vi "Magnet Gap Tester (RT).vi"() -> ()   [LabVIEW 2013]
uses:
  Controls/i2c_state.ctl
  Controls/Host_I2CBus_Options.ctl
  Controls/i2c_Protocol_Timing.ctl
  <vilib>/Analysis/polynomials.llb/Scalar Polynomial Evaluation (DBL).vi
  <vilib>/Utility/error.llb/Error Cluster From Error Code.vi
  <vilib>/rvi/errors/niLvFpgaAdjustHostInterfaceError.vi
  <vilib>/Analysis/polynomials.llb/1D Polynomial Evaluation (DBL).vi
  <vilib>/rvi/interface/common/niFpgaWaitOnOcc.vi
  <userlib>/_MGI/1D Array/MGI Average/MGI Average (DBL[]).vi
  <vilib>/rvi/interface/nirviReadWriteControl/nirviReadWriteControl.xnode
  Controls/FPGA_Reference.ctl
  FPGA Bitfiles/TIsbRIO_FPGATarget_TISensoredBLDC(F_DyXSZt47tvg.lvbitx
  FPGA/TI Sensored BLDC (FPGA).vi
  <vilib>/rvi/interface/nirviMethod/nirviMethod.xnode
  <vilib>/rvi/errors/niLvFpgaMergeErrorWithErrorCode.vi
  <vilib>/Analysis/NI_AALPro.lvlib
  <vilib>/FPGAPlugInAG/sbRIO-9626/niLvFpga_ReadFifo_sbRIO-9626.vi
  NiFpgaLv.dll
panel:
  out "Re-Cal (Hall)":dbl[](array[numeric])
  out "Re-Cal (Encoder)":dbl[](array[numeric])
  out "FWD Accuracy (%)":dbl
  out "REV Accuracy (%)":dbl
  out "REV Non-Linearity (%)":dbl=0.15612299232428833
  out "FWD Non-Linearity (%)":dbl=0.23166191431116404
  out "Max Hysteresis (%)":dbl=1.342957067692166
  out "Average Hysteresis (%)":dbl=0.6751303305956703
  out "Magnetic Field":u16=445
  out "Hall Pos (deg)":dbl=250.14822489420567
  out "ENC Pos (deg)":dbl=251.61773088654434
  in  "Motor Stop Offset":i32
  in  "REV Limit":dbl=90.0
  in  "FWD Limit":dbl=270.0
  out "XY Graph":cluster{dbl[], dbl[]}[](graph)=[{array[264 elements], array[264 elements]}, {array[264 elements], array[264 elements]}, {array[3405 elements], array[3405 elements]}, {array[3405 elements], array[3405 elements]}, {array[3405 elements], array[3405 elements]}, {[15041.030640668523, 5013.676880222842], [15041.030640668523, 5013.676880222842]}]
  out "Hall Elements":u32=3405
  out "Encoder Elements":u32=3405
  out "REV OUT":bool
  out "FWD OUT":bool
  in  "Reverse":bool
  in  "Forward":bool
  out "AI0":fxp<+/-,24,5>=2.0473861694335938
  out "ENC Pos (Counts)":i32=14017
  out "AI Loop Actual":u32=17
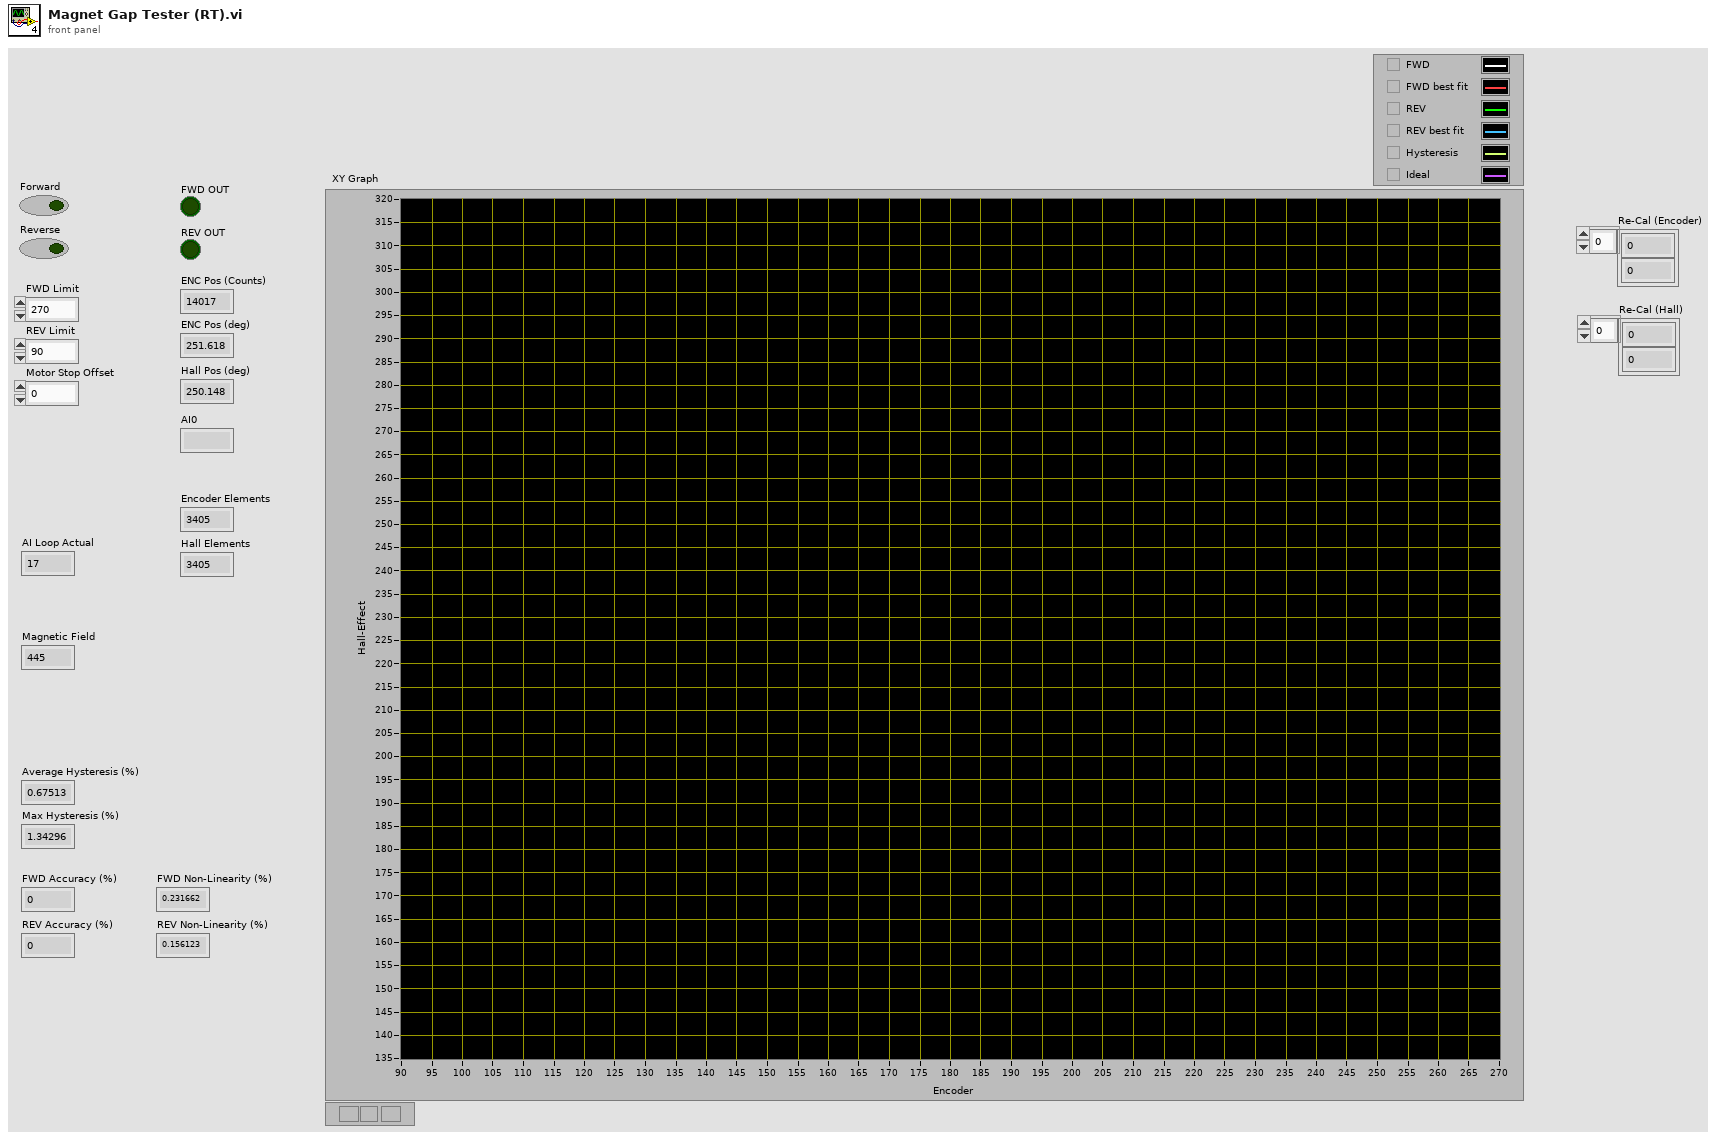
[diagram p1: front panel]
types:
  T1 = typedef "i2c_Protocol_Timing.ctl" = cluster{"SCL Period (Ticks)":u32, "TransmitDelay(Ticks)":u32, "PostAddressDelay(Ticks)":u32, "StartStopDelay(Ticks)":u32}
  T2 = typedef "Host_I2CBus_Options.ctl" = enum16{"Open I2C Bus", "Send CMD", "Close I2C Bus"}
  T3 = typedef "i2c_state.ctl" = enum16{"Monitor", "W_To_Device", "R_From_Device", "W/R_From_Device", "TerminateCore"}
  T4 = cluster{"Use_10-Bit_Address":bool, "Slave Device Address":u8, "10-Bit_Address":u8, "NumBytesToRead":i32, "i2c Core Option":T3}
  T5 = typedef "FPGA_Reference.ctl" = refnum<k20>
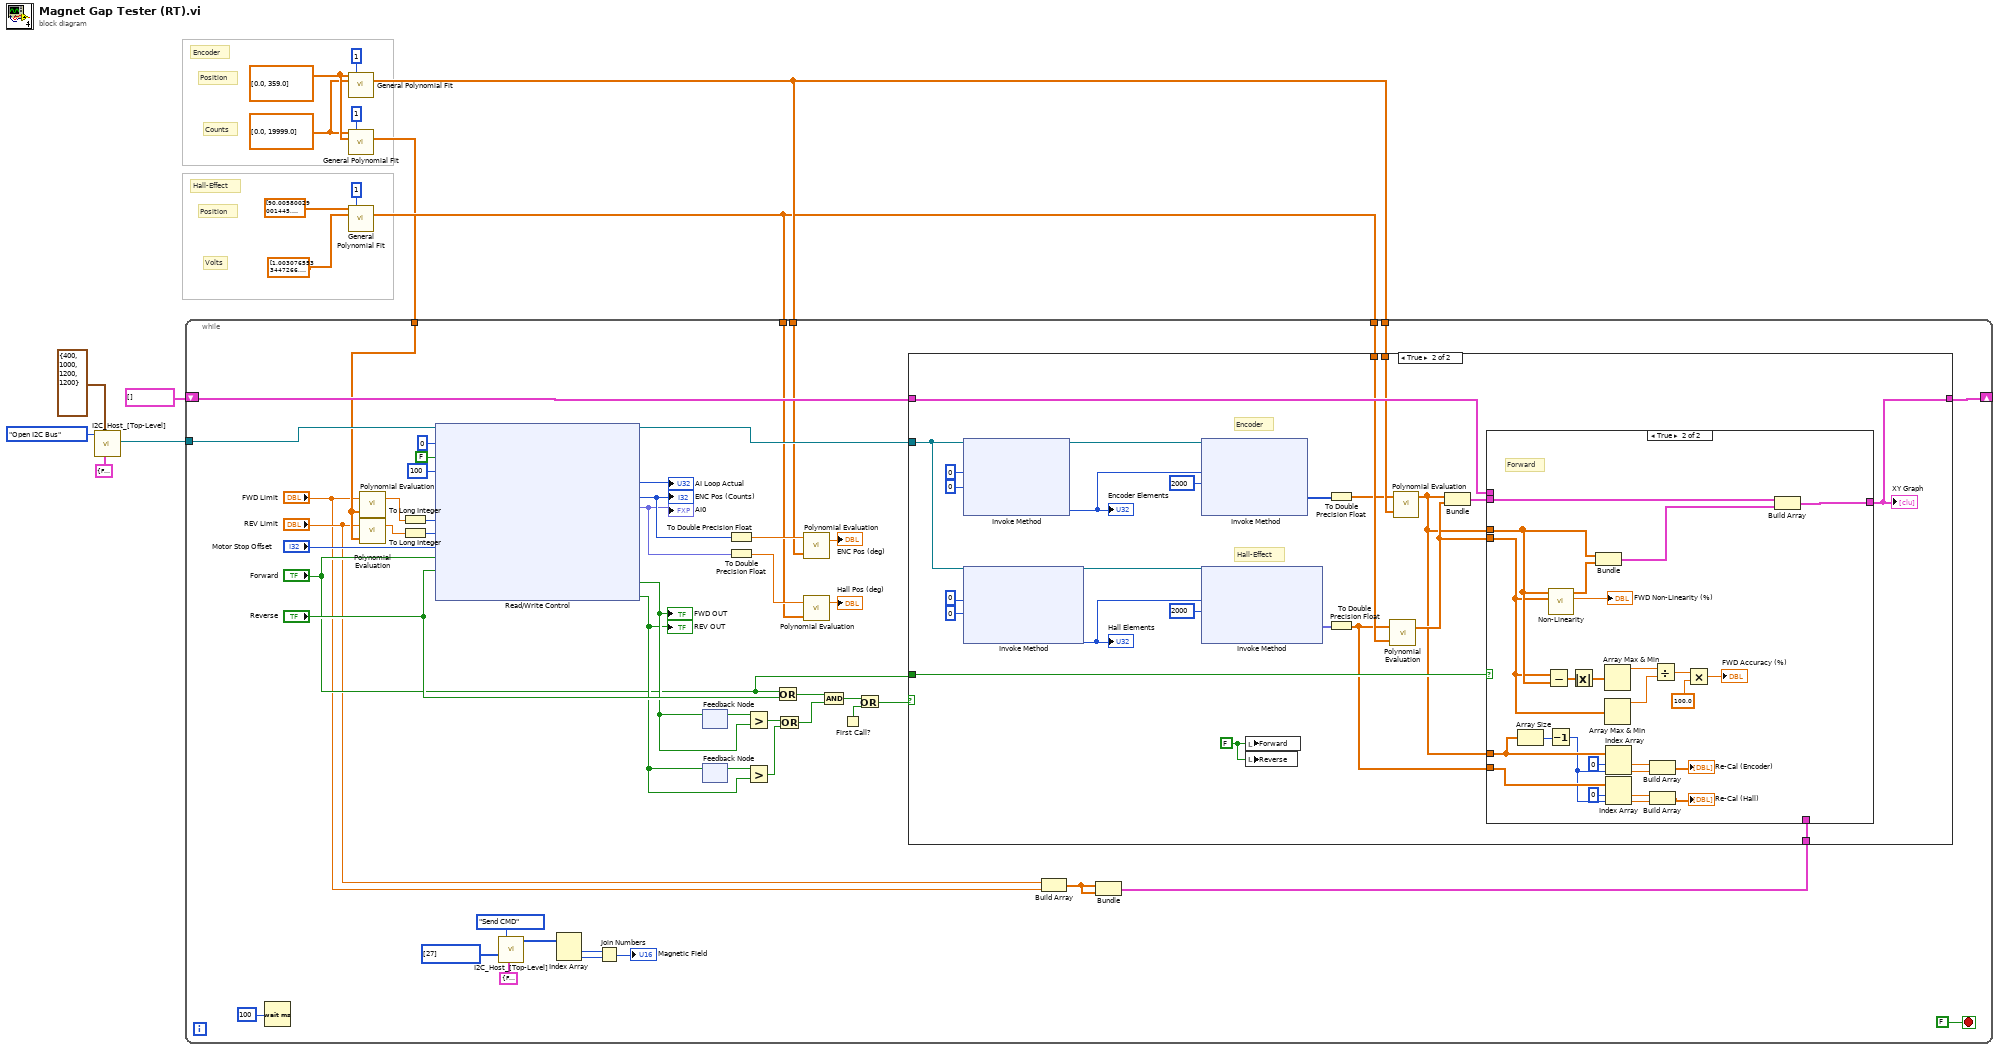
[diagram p0: block diagram]
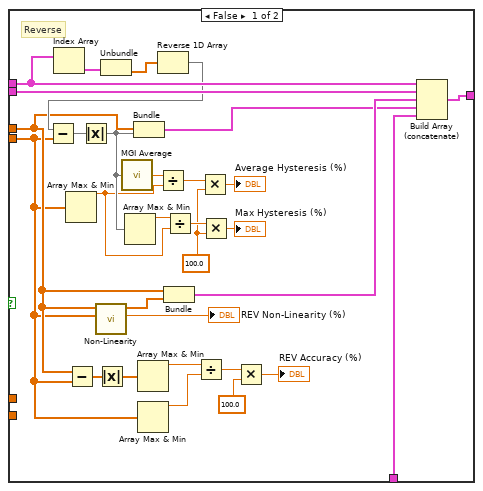
[diagram p3: hidden frame]
diagram:
  w4 = dbl[] [0.0, 19999.0] ("Y")
  w5 = dbl[] [0.0, 359.0] ("Y")
  # "Hall-Effect"
  # "Position"
  # "Volts"
  # "Encoder"
  # "Position"
  # "Counts"
  n1 = call "I2C_Host_[Top-Level].vi"("I2C Parameters"=T4 {"Use_10-Bit_Address"=FALSE, "Slave Device Address"=208, "10-Bit_Address"=0, "NumBytesToRead"=1, "i2c Core Option"=enum."W/R_From_Device"}, "Protocol_Timing"=T1 {"SCL Period (Ticks)"=400, "TransmitDelay(Ticks)"=1000, "PostAddressDelay(Ticks)"=1200, "StartStopDelay(Ticks)"=1200}, "I2C Bus"=Host_I2CBus_Options."Open I2C Bus") -> ("FPGA VI Reference Out"=w10:T5)  [unwired: 5 in, 3 out]
  n2 = call <vilib>:"General Polynomial Fit.vi"("Y"=w5, "polynomial order"=1, "X"=w4) -> ("Polynomial Coefficients"=w13:dbl[])  [unwired: 9 in, 3 out]
  n3 = call <vilib>:"General Polynomial Fit.vi"("Y"=w4, "polynomial order"=1, "X"=w5) -> ("Polynomial Coefficients"=w3:dbl[])  [unwired: 9 in, 3 out]
  n4 = call <vilib>:"General Polynomial Fit.vi"("Y"=dbl[] [90.00580029001445, 269.9814990749538] ("Re-Cal (Encoder)"), "polynomial order"=1, "X"=dbl[] [1.0030765533447266, 2.652881622314453] ("Re-Cal (Hall)")) -> ("Polynomial Coefficients"=w11:dbl[])  [unwired: 9 in, 3 out]
  n5 = while {
    tunnel: w10 -> [w64]
    shift-right: [w44] -> _
    shift-left: cluster{dbl[], dbl[]}[] [] -> [w46]
    tunnel: w13 -> [w40]
    tunnel: w13 -> [w38]
    tunnel: w11 -> [w37]
    tunnel: w11 -> [w35]
    tunnel: w3 -> [w22]
    stop <- FALSE stop-if-true
    n6 = Wait (ms)(milliseconds to wait=u32 100) -> ()  [unwired: 1 out]
    n7 = call-poly <vilib>:"Polynomial Evaluation.vi"("P(x)"=w22, "a"="FWD Limit") -> ("P(a)"=w20:dbl)  [unwired: 1 out]
    n8 = call-poly <vilib>:"Polynomial Evaluation.vi"("P(x)"=w22, "a"="REV Limit") -> ("P(a)"=w21:dbl)  [unwired: 1 out]
    n9 = To Long Integer(number=w20) -> (32bit integer=w24:i32)
    n10 = To Long Integer(number=w21) -> (32bit integer=w23:i32)
    n11 = xnode "Read/Write Control"("FPGA VI Reference In"=w64, "AI Loop (uSec)"=u32 0, "Position Reset"=FALSE, "Samples to Avg"=i16 100, "FWD Limit"=w24, "REV Limit"=w23, "Motor Stop Offset"="Motor Stop Offset", "Forward"="Forward", "Reverse"="Reverse") -> ("FPGA VI Reference Out"=w59:T5, "AI Loop Actual"=→"AI Loop Actual":u32, "Position (Counts)"=w42:i32, "AI0 (avg)"=w31:fxp<+/-,24,5>, "FWD OUT"=w55:bool, "REV OUT"=w53:bool)  [unwired: 1 in, 1 out]
    "ENC Pos (Counts)" <- w42
    "AI0" <- w31
    "FWD OUT" <- w55
    "REV OUT" <- w53
    n12 = call "I2C_Host_[Top-Level].vi"("CMD_Bytes"=u8[] [27], "I2C Parameters"=T4 {"Use_10-Bit_Address"=FALSE, "Slave Device Address"=108, "10-Bit_Address"=0, "NumBytesToRead"=2, "i2c Core Option"=enum."W/R_From_Device"}, "I2C Bus"=Host_I2CBus_Options."Send CMD") -> ("DataBytes"=w29:u8[])  [unwired: 5 in, 3 out]
    n13 = Index Array(array=w29) -> (element #1=w28:u8, element #2=w27:u8)  [unwired: 2 in]
    n14 = Join Numbers(hi=w28, lo=w27) -> ((hi.lo)=→"Magnetic Field":u16)
    n15 = feedback-in #1(w55) -> ()
    n16 = feedback #1() -> (w56:bool)  [unwired: 1 in]
    n17 = feedback #2() -> (w54:bool)  [unwired: 1 in]
    n18 = feedback-in #2(w53) -> ()
    n19 = To Double Precision Float(number=w42) -> (double precision float=w41:dbl)
    n20 = To Double Precision Float(number=w31) -> (double precision float=w36:dbl)
    n21 = Greater?(x=w56, y=w55) -> (0:w52:bool)
    n22 = Greater?(x=w54, y=w53) -> (0:w51:bool)
    n23 = Or(x="Forward", y="Reverse") -> (x .or. y?=w45:bool)
    n24 = Or(x=w52, y=w51) -> (x .or. y?=w50:bool)
    n25 = call-poly <vilib>:"Polynomial Evaluation.vi"("P(x)"=w40, "a"=w41) -> ("P(a)"=→"ENC Pos (deg)":dbl)  [unwired: 1 out]
    n26 = call-poly <vilib>:"Polynomial Evaluation.vi"("P(x)"=w35, "a"=w36) -> ("P(a)"=→"Hall Pos (deg)":dbl)  [unwired: 1 out]
    n27 = And(x=w45, y=w50) -> (x .and. y?=w49:bool)
    n28 = First Call?() -> (First Call?: T/F=w48:bool)
    n29 = Or(x=w49, y=w48) -> (x .or. y?=w47:bool)
    n30 = Build Array("REV Limit", "FWD Limit") -> (w19:dbl[])
    n31 = Bundle(w19, w19) -> (w18:cluster{dbl[], dbl[]})  [unwired: 1 in]
    n32 = case shown="True" w47 {
      tunnel: w59 -> [_ w90]
      tunnel: w46 -> [w66 w76]
      tunnel: "Forward" -> [_ w78]
      tunnel: [w66 w75] -> w44
      tunnel: w38 -> [_ w73]
      tunnel: w37 -> [_ w72]
      tunnel: w18 -> [_ w70]
      frame False {
      }
      frame True {
        w79 = FALSE ("Forward")
        # "Hall-Effect"
        # "Encoder"
        n33 = xnode "Invoke Method"("FPGA VI Reference In"=w90, "Number of Elements"=u32 0, "Timeout (ms)"=0) -> ("FPGA VI Reference Out"=w91:T5, "Elements Remaining"=w84:u32)  [unwired: 1 in, 2 out]
        "Encoder Elements" <- w84
        n34 = xnode "Invoke Method"("FPGA VI Reference In"=w90, "Number of Elements"=u32 0, "Timeout (ms)"=0) -> ("FPGA VI Reference Out"=w89:T5, "Elements Remaining"=w83:u32)  [unwired: 1 in, 2 out]
        "Hall Elements" <- w83
        n35 = xnode "Invoke Method"("FPGA VI Reference In"=w91, "Number of Elements"=w84, "Timeout (ms)"=2000) -> ("Data"=w74:i32[])  [unwired: 1 in, 3 out]
        n36 = xnode "Invoke Method"("FPGA VI Reference In"=w89, "Number of Elements"=w83, "Timeout (ms)"=2000) -> ("Data"=w82:fxp<+/-,24,5>[])  [unwired: 1 in, 3 out]
        n37 = local write "Forward"(w79) -> ()
        n38 = local write "Reverse"(w79) -> ()
        n39 = To Double Precision Float(number=w74) -> (double precision float=w69:dbl[])
        n40 = To Double Precision Float(number=w82) -> (double precision float=w68:dbl[])
        n41 = call-poly <vilib>:"Polynomial Evaluation.vi"("P(x)"=w72, "A"=w68) -> ("P(A)"=w71:dbl[])  [unwired: 1 out]
        n42 = call-poly <vilib>:"Polynomial Evaluation.vi"("P(x)"=w73, "A"=w69) -> ("P(A)"=w67:dbl[])  [unwired: 1 out]
        n43 = Bundle("P(A)"=w67, "P(A)"=w71) -> (w77:cluster{"P(A)":dbl[], "P(A)":dbl[]})  [unwired: 1 in]
        n44 = case shown="True" w78 {
          tunnel: w77 -> [w121 w147]
          tunnel: [w120 w146] -> w75
          tunnel: w76 -> [w104 _]
          tunnel: w67 -> [w99 w135]
          tunnel: w71 -> [w98 w134]
          tunnel: w70 -> [w105 _]
          tunnel: w67 -> [_ w133]
          tunnel: w68 -> [_ w132]
          frame False {
            w108 = 100.0 ("y")
            # "Reverse"
            n45 = Index Array(array=w104) -> (element=w103:cluster{dbl[], dbl[]})  [unwired: 1 in]
            n46 = Array Max & Min(array=w98) -> (max value=w111:dbl)  [unwired: 3 out]
            n47 = Subtract(x=w99, y=w98) -> (x-y=w100:dbl[])
            n48 = call "Non-Linearity.vi"("Hall-Effect"=w98, "Encoder"=w99) -> ("Non-Linearity (%)"=→"REV Non-Linearity (%)":dbl, "Best Linear Fit"=w117:dbl[])  [unwired: 8 in]
            n49 = Absolute Value(x=w100) -> (abs(x)=w96:dbl[])
            n50 = Unbundle(w103) -> (w102:dbl[])  [unwired: 1 out]
            n51 = Array Max & Min(array=w96) -> (max value=w95:dbl)  [unwired: 3 out]
            n52 = Array Max & Min(array=w98) -> (max value=w94:dbl)  [unwired: 3 out]
            n53 = Reverse 1D Array(array=w102) -> (reversed array=w101:dbl[])
            n54 = Subtract(x=w101, y=w98) -> (x-y=w119:dbl[])
            n55 = Absolute Value(x=w119) -> (abs(x)=w118:dbl[])
            n56 = call-poly <userlib>:"MGI Average.vi"("Double[]"=w118) -> ("Average"=w113:dbl)  [unwired: 1 in]
            n57 = Array Max & Min(array=w118) -> (max value=w112:dbl)  [unwired: 3 out]
            n58 = Bundle("P(A)"=w99, w118) -> (w114:cluster{"P(A)":dbl[], dbl[]})  [unwired: 1 in]
            n59 = Divide(x=w113, y=w111) -> (x/y=w110:dbl)
            n60 = Bundle("P(A)"=w99, "Best Linear Fit"=w117) -> (w115:cluster{"P(A)":dbl[], "Best Linear Fit":dbl[]})  [unwired: 1 in]
            n61 = Divide(x=w112, y=w111) -> (x/y=w109:dbl)
            n62 = Divide(x=w95, y=w94) -> (x/y=w93:dbl)
            n63 = Multiply(x=w110, y=w108) -> (x*y=→"Average Hysteresis (%)":dbl)
            n64 = Multiply(x=w109, y=w108) -> (x*y=→"Max Hysteresis (%)":dbl)
            n65 = Multiply(x=w93, y=100.0) -> (x*y=→"REV Accuracy (%)":dbl)
            n66 = Build Array (concatenate)(w104, w121, w115, w114, w105) -> (w120:cluster{"P(A)":dbl[], "Best Linear Fit":dbl[]}[])
          }
          frame True {
            # "Forward"
            n67 = Array Size(array=w133) -> (size(s)=w129:i32)
            n68 = Subtract(x=w134, y=w135) -> (x-y=w142:dbl[])
            n69 = Decrement(x=w129) -> (x-1=w128:i32)
            n70 = call "Non-Linearity.vi"("Hall-Effect"=w134, "Encoder"=w135) -> ("Non-Linearity (%)"=→"FWD Non-Linearity (%)":dbl, "Best Linear Fit"=w144:dbl[])  [unwired: 8 in]
            n71 = Absolute Value(x=w142) -> (abs(x)=w140:dbl[])
            n72 = Bundle("P(A)"=w135, "Best Linear Fit"=w144) -> (w145:cluster{"P(A)":dbl[], "Best Linear Fit":dbl[]})  [unwired: 1 in]
            n73 = Array Max & Min(array=w140) -> (max value=w139:dbl)  [unwired: 3 out]
            n74 = Array Max & Min(array=w134) -> (max value=w138:dbl)  [unwired: 3 out]
            n75 = Index Array(array=w133, index #1=0 ("index"), index #2=w128) -> (element #1=w127:dbl, element #2=w126:dbl)
            n76 = Index Array(array=w132, index #1=0 ("index"), index #2=w128) -> (element #1=w125:dbl, element #2=w124:dbl)
            n77 = Build Array(w127, w126) -> (→"Re-Cal (Encoder)":dbl[])
            n78 = Build Array(w125, w124) -> (→"Re-Cal (Hall)":dbl[])
            n79 = Divide(x=w139, y=w138) -> (x/y=w137:dbl)
            n80 = Multiply(x=w137, y=100.0) -> (x*y=→"FWD Accuracy (%)":dbl)
            n81 = Build Array(w147, w145) -> (w146:cluster{"P(A)":dbl[], "Best Linear Fit":dbl[]}[])
          }
        }
        "XY Graph" <- w75
      }
    }
  }
